vi "channelcontrolsub.vi"(0 "TorqueSample":dbl, 1 "dt":dbl, 3 "Limit Number":dbl, 4 "Torque":bool, 5 "ControlPara":dbl[](array[numeric]), 7 "AngleSample":dbl, 8 "Angel":bool, 9 "syn-angel":dbl, 12 "Command":dbl, 15 "TempAngle":dbl, 16 "output range":cluster{"output high":dbl, "output low":dbl}, 17 "ChannelStatus":T1 items=["通道关", "位置通道", "加载通道"]) -> (19 "syn out":dbl, 20 "output":dbl, 21 "syn-angle":dbl, 22 "forward":dbl, 23 "TempAngleOut":dbl, 24 "diff syn out 2":dbl, 25 "control out":dbl, 27 "Commandout":dbl)   [LabVIEW 2014]
uses:
  Control 1.ctl
  <vilib>/addons/control/pid/pid.llb/PID (DBL).vi
  <vilib>/addons/control/pid/pid.llb/PID Lead-Lag (DBL).vi
  <vilib>/addons/control/pid/NI_PID_pid.lvlib
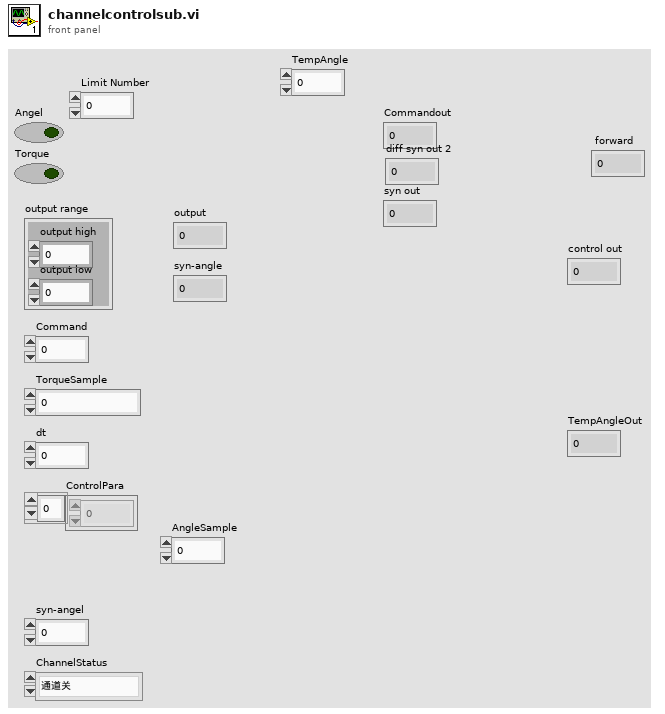
[diagram p1: front panel]
types:
  T1 = typedef "Control 1.ctl" = i32
  T2 = cluster{"gain":dbl, "lag time":dbl, "lead time":dbl}
  T3 = cluster{"Numeric":dbl, "Numeric":dbl, "Numeric":dbl}
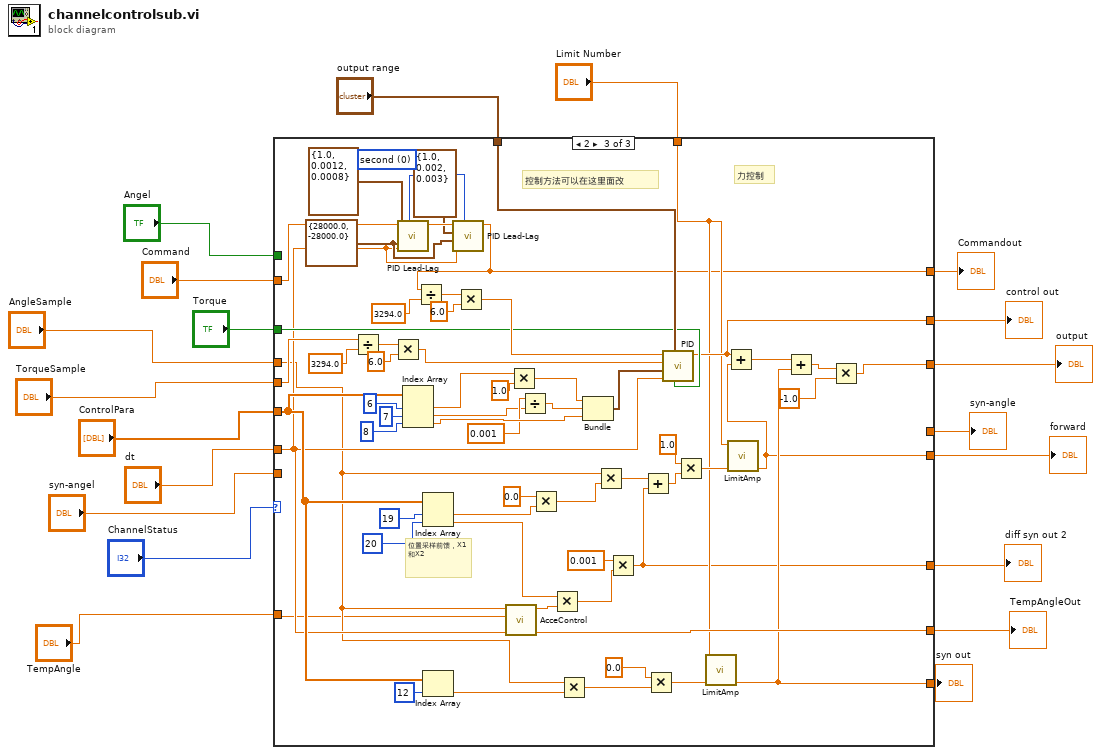
[diagram p0: block diagram]
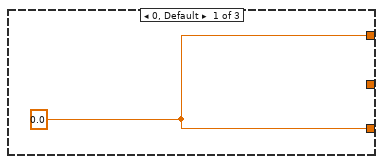
[diagram p2: hidden frame]
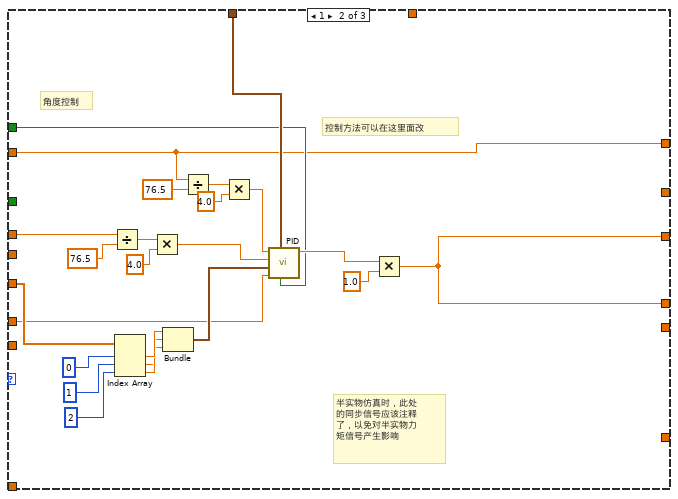
[diagram p3: hidden frame]
diagram:
  n1 = case shown="2" "ChannelStatus" {
    tunnel: "dt" -> [_ w30 w53]
    tunnel: "output range" -> [_ w27 w106]
    tunnel: "Command" -> [_ w22 w58]
    tunnel: "ControlPara" -> [_ w42 w72]
    tunnel: [w21 w25 w64] -> w19
    tunnel: "TorqueSample" -> [_ _ w91]
    tunnel: "syn-angel" -> [_ _ _]
    tunnel: [_ w25 _] -> w20
    tunnel: "AngleSample" -> [_ w24 w49]
    tunnel: "Angel" -> [_ w23 _]
    tunnel: "Torque" -> [_ _ w90]
    tunnel: [w21 w22 w54] -> w10
    tunnel: "TempAngle" -> [_ _ w46]
    tunnel: [_ _ w84] -> w9
    tunnel: [_ _ w74] -> w8
    tunnel: "Limit Number" -> [_ _ w68]
    tunnel: [_ _ w48] -> w6
    tunnel: [_ _ w66] -> w5
    tunnel: [_ _ w65] -> w4
    frame 0, Default {
      w21 = 0.0 ("output")
    }
    frame 1 {
      # "半实物仿真时，此处\n的同步信号应该注释\n了，以免对半实物力\n矩信号产生影响"
      # "控制方法可以在这里面改"
      # "角度控制"
      n2 = Divide(x=w24, y=76.5) -> (x/y=w36:dbl)
      n3 = Index Array(array=w42, index #1=0 ("index"), index #2=1 ("index"), index #3=2 ("index")) -> (element #1=w34:dbl, element #2=w26:dbl, element #3=w33:dbl)
      n4 = Multiply(x=w36, y=4.0) -> (x*y=w29:dbl)
      n5 = Bundle("Numeric"=w34, "Numeric"=w26, "Numeric"=w33) -> (w31:T3)  [unwired: 1 in]
      n6 = Divide(x=w22, y=76.5) -> (x/y=w39:dbl)
      n7 = Multiply(x=w39, y=4.0) -> (x*y=w28:dbl)
      n8 = call-poly <vilib>:"PID.vi"("reinitialize? (F)"=w23, "output range"=w27, "dt (s)"=w30, "PID gains"=w31, "process variable"=w29, "setpoint"=w28) -> ("output"=w32:dbl)  [unwired: 4 in, 1 out]
      n9 = Multiply(x=w32, y=1.0) -> (x*y=w25:dbl)
    }
    frame 2 {
      w55 = cluster{"output high":dbl, "output low":dbl} {"output high"=28000.0, "output low"=-28000.0} ("output range")
      w51 = u16 0 items=["second", "minute"] ("time unit")
      # "位置采样前馈，X1和X2"
      # "力控制"
      # "控制方法可以在这里面改"
      n10 = Divide(x=w91, y=3294.0) -> (x/y=w95:dbl)
      n11 = Multiply(x=w95, y=6.0) -> (x*y=w94:dbl)
      n12 = call-poly <vilib>:"PID Lead-Lag.vi"("time unit"=w51, "dt (s)"=w53, "output range"=w55, "tuning parameters"=T2 {"gain"=1.0, "lag time"=0.0012, "lead time"=0.0008}, "input"=w58) -> ("output"=w56:dbl)  [unwired: 3 in, 1 out]
      n13 = Index Array(array=w72, index #1=6 ("index"), index #2=7 ("index"), index #3=8 ("index")) -> (element #1=w61:dbl, element #2=w59:dbl, element #3=w93:dbl)
      n14 = Index Array(array=w72, index #1=19 ("index"), index #2=20 ("index")) -> (element #1=w76:dbl, element #2=w47:dbl)
      n15 = Index Array(array=w72, index=12) -> (element=w50:dbl)
      n16 = call-poly <vilib>:"PID Lead-Lag.vi"("time unit"=w51, "dt (s)"=w53, "output range"=w55, "tuning parameters"=T2 {"gain"=1.0, "lag time"=0.002, "lead time"=0.003}, "input"=w56) -> ("output"=w54:dbl)  [unwired: 3 in, 1 out]
      n17 = Divide(x=w54, y=3294.0) -> (x/y=w99:dbl)
      n18 = Multiply(x=w99, y=6.0) -> (x*y=w98:dbl)
      n19 = call "AcceControl.vi"("dt"=w53, "TempAngle"=w46, "angle sample"=w49) -> ("temp angle out"=w84:dbl, "control out"=w85:dbl)  [unwired: 7 in]
      n20 = Multiply(x=w61, y=1.0) -> (x*y=w88:dbl)
      n21 = Divide(x=0.001 ("y"), y=w59) -> (x/y=w87:dbl)
      n22 = Multiply(x=0.0 ("y"), y=w76) -> (x*y=w77:dbl)
      n23 = Multiply(x=w47, y=w85) -> (x*y=w79:dbl)
      n24 = Multiply(x=w49, y=w50) -> (x*y=w70:dbl)
      n25 = Bundle(w88, w87, "Numeric"=w93) -> (w102:cluster{dbl, dbl, "Numeric":dbl})  [unwired: 1 in]
      n26 = Multiply(x=w49, y=w77) -> (x*y=w83:dbl)
      n27 = Multiply(x=0.001 ("y"), y=w79) -> (x*y=w65:dbl)
      n28 = Add(x=w83, y=w65) -> (x+y=w82:dbl)
      n29 = Multiply(x=0.0 ("y"), y=w70) -> (x*y=w69:dbl)
      n30 = call-poly <vilib>:"PID.vi"("reinitialize? (F)"=w90, "output range"=w106, "dt (s)"=w53, "PID gains"=w102, "process variable"=w94, "setpoint"=w98) -> ("output"=w74:dbl)  [unwired: 4 in, 1 out]
      n31 = Multiply(x=1.0 ("y"), y=w82) -> (x*y=w75:dbl)
      n32 = call "LimitAmp.vi"("data in"=w69, "limit"=w68) -> ("data out"=w66:dbl)  [unwired: 9 in]
      n33 = call "LimitAmp.vi"("data in"=w75, "limit"=w68) -> ("data out"=w48:dbl)  [unwired: 9 in]
      n34 = Add(x=w74, y=w48) -> (x+y=w67:dbl)
      n35 = Add(x=w67, y=w66) -> (x+y=w63:dbl)
      n36 = Multiply(x=w63, y=-1.0) -> (x*y=w64:dbl)
    }
  }
  "syn-angle" <- w20
  "output" <- w19
  "Commandout" <- w10
  "syn out" <- w5
  "TempAngleOut" <- w9
  "control out" <- w8
  "forward" <- w6
  "diff syn out 2" <- w4
